vi "Pre Launch Init.vi"(11 "CS++StartActor in":refnum<class "CS++StartActor.lvclass">) -> (0 "error out":errorcluster, 3 "CS++StartActor out":refnum<class "CS++StartActor.lvclass">)   [LabVIEW 2012, in "CS++StartActor.lvlib" / "CS++StartActor.lvclass"]
doc: "(<B>Filename</B>: Actor Framework.lvlib:Actor.lvclass:Pre Launch Init.vi)\n\nDefines behavior that occurs after the Launch Actor method is invoked but before the actor's Actor Core method begins running.\n\nThe Pre Launch Init method is guaranteed to finish before the Launch Actor method returns to its caller and before the actor itself receives any messages. Any references that the Pre Launch Init method obtains are guaranteed to have the same lifetime as the actor itself. Any errors that the Pre Launch Init method returns will abort the launch.\n\nBy default, this method does nothing. A descendant class may override it to define behavior."
uses:
  CS++StartActor.lvclass
  CS++StartActor.lvclass/CS++StartActor.ctl
  CS++BaseActor/CS++BaseActor.lvclass
  Libraries/MessageLogger/CS++MessageLogger.lvlib
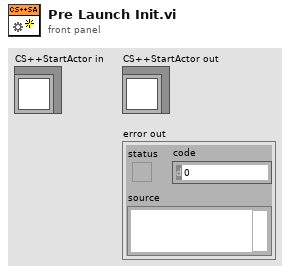
[diagram p1: front panel]
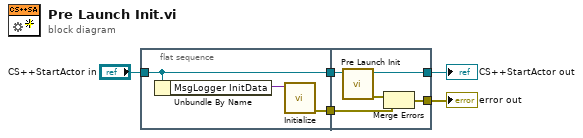
[diagram p0: block diagram]
diagram:
  n1 = flat-sequence {
    tunnel: "CS++StartActor in" -> [w7]
    tunnel: [w7] -> w2
    tunnel: [w6] -> w1
    tunnel: [w10] -> w5
    tunnel: [w12] -> w4
    tunnel: w2 -> [w11]
    tunnel: w1 -> [w9]
    frame #0 {
      n2 = Unbundle By Name(w7) -> ("MsgLogger InitData"=w8:variant)
      n3 = call "Initialize.vi"("Initialization Data"=w8) -> ("Error Out"=w6:errorcluster)  [unwired: 10 in]
    }
    frame #1 {
      n4 = call-parent "Pre Launch Init.vi"("CS++BaseActor in"=w11) -> ("error out"=w13:errorcluster, "CS++BaseActor out"=w12:refnum<class "CS++StartActor.lvclass">)  [unwired: 9 in]
      n5 = Merge Errors(w13, w9) -> (w10:errorcluster)
    }
  }
  "error out" <- w5
  "CS++StartActor out" <- w4
